vi "test-swerve-drve-odometry-02.vi"() -> (3 "Test Passed":bool)   [LabVIEW 2019]
uses:
  <vilib>/Rock Robotics/WPI/ThirdParty/JAS_Junk/TrajLib/TypeDef/SWERVE_DRIVE_ODOMETRY.ctl
  <vilib>/Rock Robotics/WPI/ThirdParty/JAS_Junk/TrajLib/TypeDef/POSE2D.ctl
  <vilib>/Rock Robotics/WPI/ThirdParty/JAS_Junk/TrajLib/TypeDef/TRANSLATION2D.ctl
  <vilib>/Rock Robotics/WPI/ThirdParty/JAS_Junk/TrajLib/TypeDef/ROTATION2D.ctl
  <vilib>/Rock Robotics/WPI/ThirdParty/JAS_Junk/TrajLib/TypeDef/SWERVE_DRIVE_MODULE_POSITION.ctl
  <vilib>/Rock Robotics/WPI/ThirdParty/JAS_Junk/TrajLib/TypeDef/SWERVE_DRIVE_KINEMATICS.ctl
  <vilib>/Analysis/Matrix/Datatypes/RealMatrix.ctl
  <vilib>/Rock Robotics/WPI/ThirdParty/JAS_Junk/TrajLib/TypeDef/SWERVE_DRIVE_MODULE_STATE.ctl
  <vilib>/Rock Robotics/WPI/ThirdParty/JAS_Junk/TrajLib/Conv_Deg_Radians.vi
  <vilib>/Rock Robotics/WPI/ThirdParty/JAS_Junk/TrajLib/Rotation2d_CreateAngle.vi
  <vilib>/Rock Robotics/WPI/ThirdParty/JAS_Junk/TrajLib/Trajectory_Library.lvlib
  <vilib>/Analysis/Matrix/NI_Matrix.lvlib
panel:
  out "SWERVE_DRIVE_KINEMATICS":T1 {"SavedModuleStates"."Angle"."SIN" format="%13.4f"; "SavedModuleStates"."Angle"."COS" format="%13.4f"; "SavedModuleStates"."Angle"."VALUE" format="%13.4f"; "PrevCoR"."Y" format="%14.3f"; "PrevCoR"."X" format="%14.3f"; "Modules"."Y" format="%14.3f"; "Modules"."X" format="%14.3f"}
  out "Odom 1":T6={"POSE"={"TRANSLATION"={"X"=0.0, "Y"=0.0}, "ROTATION"={"VALUE"=0.0, "COS"=1.0, "SIN"=0.0}}, "GyroOffset"={"VALUE"=0.0, "COS"=1.0, "SIN"=0.0}, "PreviousAngle"={"VALUE"=0.0, "COS"=1.0, "SIN"=0.0}, "PrevModulePositions"=[], "NumModules"=0} {"PrevModulePositions"."Angle"."SIN" format="%13.4f"; "PrevModulePositions"."Angle"."COS" format="%13.4f"; "PrevModulePositions"."Angle"."VALUE" format="%13.4f"; "PreviousAngle"."SIN" format="%13.4f"; "PreviousAngle"."COS" format="%13.4f"; "PreviousAngle"."VALUE" format="%13.4f"; "GyroOffset"."SIN" format="%13.4f"; "GyroOffset"."COS" format="%13.4f"; "GyroOffset"."VALUE" format="%13.4f"; "POSE"."ROTATION"."SIN" format="%13.4f"; "POSE"."ROTATION"."COS" format="%13.4f"; "POSE"."ROTATION"."VALUE" format="%13.4f"; "POSE"."TRANSLATION"."Y" format="%14.3f"; "POSE"."TRANSLATION"."X" format="%14.3f"}
  out "Odom 0":T6={"POSE"={"TRANSLATION"={"X"=0.0, "Y"=0.0}, "ROTATION"={"VALUE"=0.0, "COS"=1.0, "SIN"=0.0}}, "GyroOffset"={"VALUE"=0.0, "COS"=1.0, "SIN"=0.0}, "PreviousAngle"={"VALUE"=0.0, "COS"=1.0, "SIN"=0.0}, "PrevModulePositions"=[], "NumModules"=0} {"PrevModulePositions"."Angle"."SIN" format="%13.4f"; "PrevModulePositions"."Angle"."COS" format="%13.4f"; "PrevModulePositions"."Angle"."VALUE" format="%13.4f"; "PreviousAngle"."SIN" format="%13.4f"; "PreviousAngle"."COS" format="%13.4f"; "PreviousAngle"."VALUE" format="%13.4f"; "GyroOffset"."SIN" format="%13.4f"; "GyroOffset"."COS" format="%13.4f"; "GyroOffset"."VALUE" format="%13.4f"; "POSE"."ROTATION"."SIN" format="%13.4f"; "POSE"."ROTATION"."COS" format="%13.4f"; "POSE"."ROTATION"."VALUE" format="%13.4f"; "POSE"."TRANSLATION"."Y" format="%14.3f"; "POSE"."TRANSLATION"."X" format="%14.3f"}
  out "robot POSE 0":T7={"TRANSLATION"={"X"=0.0, "Y"=0.0}, "ROTATION"={"VALUE"=0.0, "COS"=1.0, "SIN"=0.0}} {"ROTATION"."SIN" format="%13.4f"; "ROTATION"."COS" format="%13.4f"; "ROTATION"."VALUE" format="%13.4f"; "TRANSLATION"."Y" format="%14.3f"; "TRANSLATION"."X" format="%14.3f"}
  out "robot POSE 1":T7={"TRANSLATION"={"X"=0.0, "Y"=0.0}, "ROTATION"={"VALUE"=0.0, "COS"=1.0, "SIN"=0.0}} {"ROTATION"."SIN" format="%13.4f"; "ROTATION"."COS" format="%13.4f"; "ROTATION"."VALUE" format="%13.4f"; "TRANSLATION"."Y" format="%14.3f"; "TRANSLATION"."X" format="%14.3f"}
  out "robot POSE 2":T7={"TRANSLATION"={"X"=0.0, "Y"=0.0}, "ROTATION"={"VALUE"=0.0, "COS"=1.0, "SIN"=0.0}} {"ROTATION"."SIN" format="%13.4f"; "ROTATION"."COS" format="%13.4f"; "ROTATION"."VALUE" format="%13.4f"; "TRANSLATION"."Y" format="%14.3f"; "TRANSLATION"."X" format="%14.3f"}
  out "Odom 2":T6={"POSE"={"TRANSLATION"={"X"=0.0, "Y"=0.0}, "ROTATION"={"VALUE"=0.0, "COS"=1.0, "SIN"=0.0}}, "GyroOffset"={"VALUE"=0.0, "COS"=1.0, "SIN"=0.0}, "PreviousAngle"={"VALUE"=0.0, "COS"=1.0, "SIN"=0.0}, "PrevModulePositions"=[], "NumModules"=0} {"PrevModulePositions"."Angle"."SIN" format="%13.4f"; "PrevModulePositions"."Angle"."COS" format="%13.4f"; "PrevModulePositions"."Angle"."VALUE" format="%13.4f"; "PreviousAngle"."SIN" format="%13.4f"; "PreviousAngle"."COS" format="%13.4f"; "PreviousAngle"."VALUE" format="%13.4f"; "GyroOffset"."SIN" format="%13.4f"; "GyroOffset"."COS" format="%13.4f"; "GyroOffset"."VALUE" format="%13.4f"; "POSE"."ROTATION"."SIN" format="%13.4f"; "POSE"."ROTATION"."COS" format="%13.4f"; "POSE"."ROTATION"."VALUE" format="%13.4f"; "POSE"."TRANSLATION"."Y" format="%14.3f"; "POSE"."TRANSLATION"."X" format="%14.3f"}
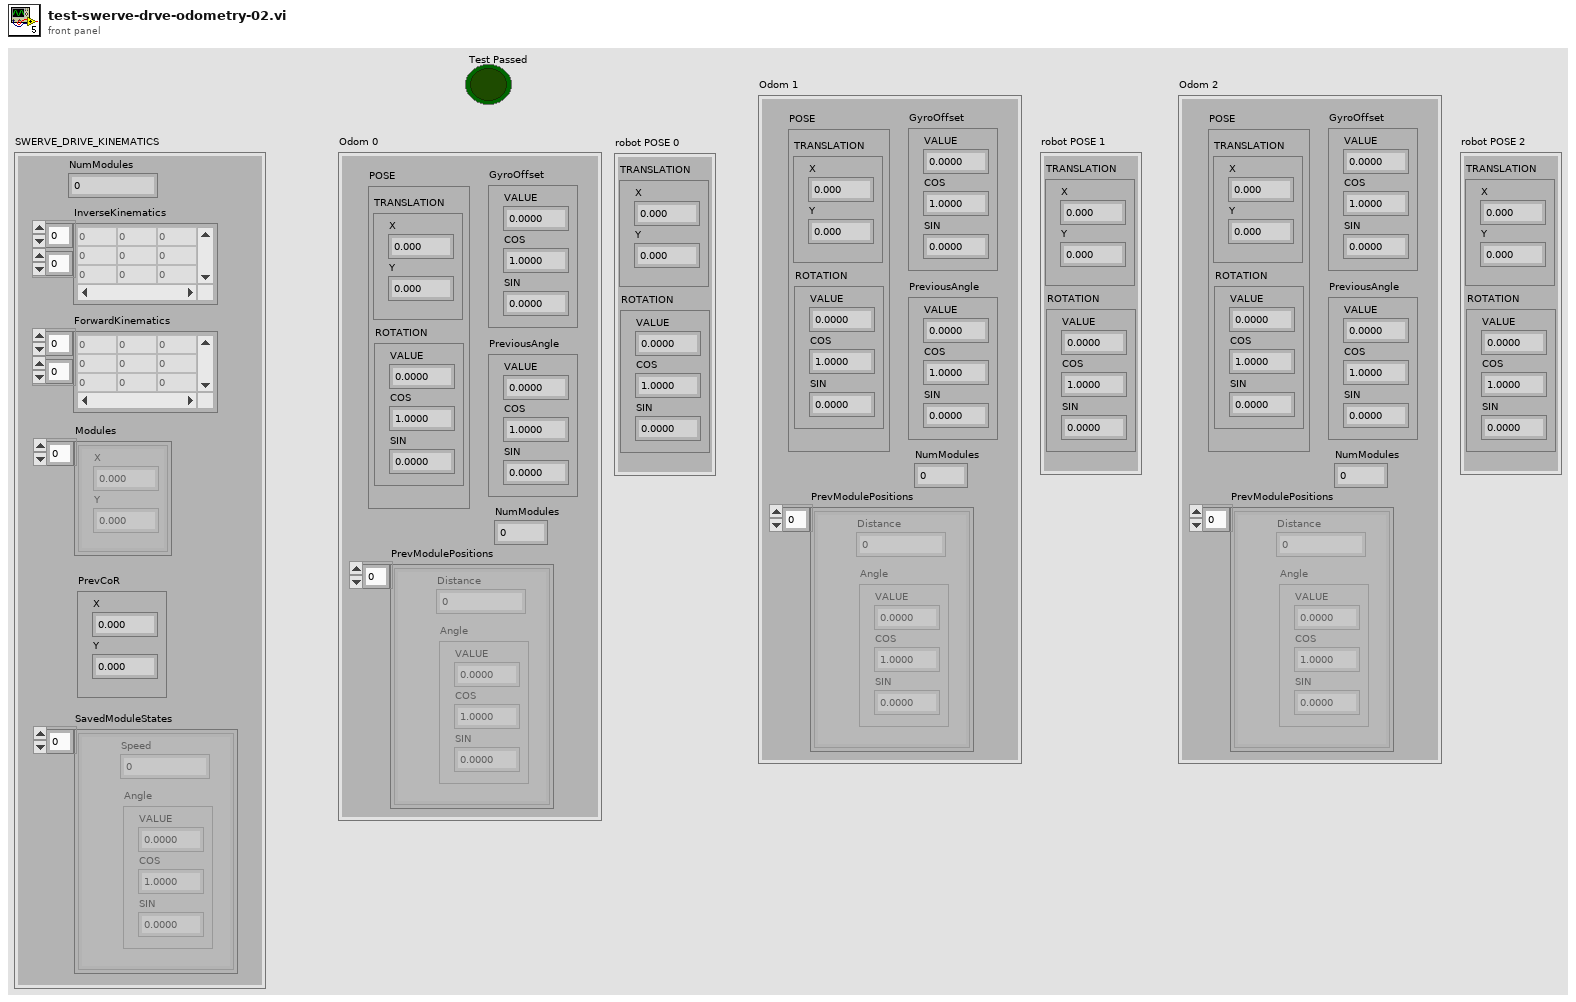
[diagram p1: front panel]
types:
  T1 = typedef "Trajectory_Library.lvlib/SWERVE_DRIVE_KINEMATICS.ctl" = cluster{"NumModules":i32, "InverseKinematics":T2, "ForwardKinematics":T2, "Modules":T3[], "PrevCoR":T3, "SavedModuleStates":T4[]}
  T2 = typedef "NI_Matrix.lvlib/RealMatrix.ctl" = dbl[][]
  T3 = typedef "Trajectory_Library.lvlib/TRANSLATION2D.ctl" = cluster{"X":dbl, "Y":dbl}
  T4 = typedef "Trajectory_Library.lvlib/SWERVE_DRIVE_MODULE_STATE.ctl" = cluster{"Speed":dbl, "Angle":T5}
  T5 = typedef "Trajectory_Library.lvlib/ROTATION2D.ctl" = cluster{"VALUE":dbl, "COS":dbl, "SIN":dbl}
  T6 = typedef "Trajectory_Library.lvlib/SWERVE_DRIVE_ODOMETRY.ctl" = cluster{"POSE":T7, "GyroOffset":T5, "PreviousAngle":T5, "PrevModulePositions":T8[], "NumModules":i32}
  T7 = typedef "Trajectory_Library.lvlib/POSE2D.ctl" = cluster{"TRANSLATION":T3, "ROTATION":T5}
  T8 = typedef "Trajectory_Library.lvlib/SWERVE_DRIVE_MODULE_POSITION.ctl" = cluster{"Distance":dbl, "Angle":T5}
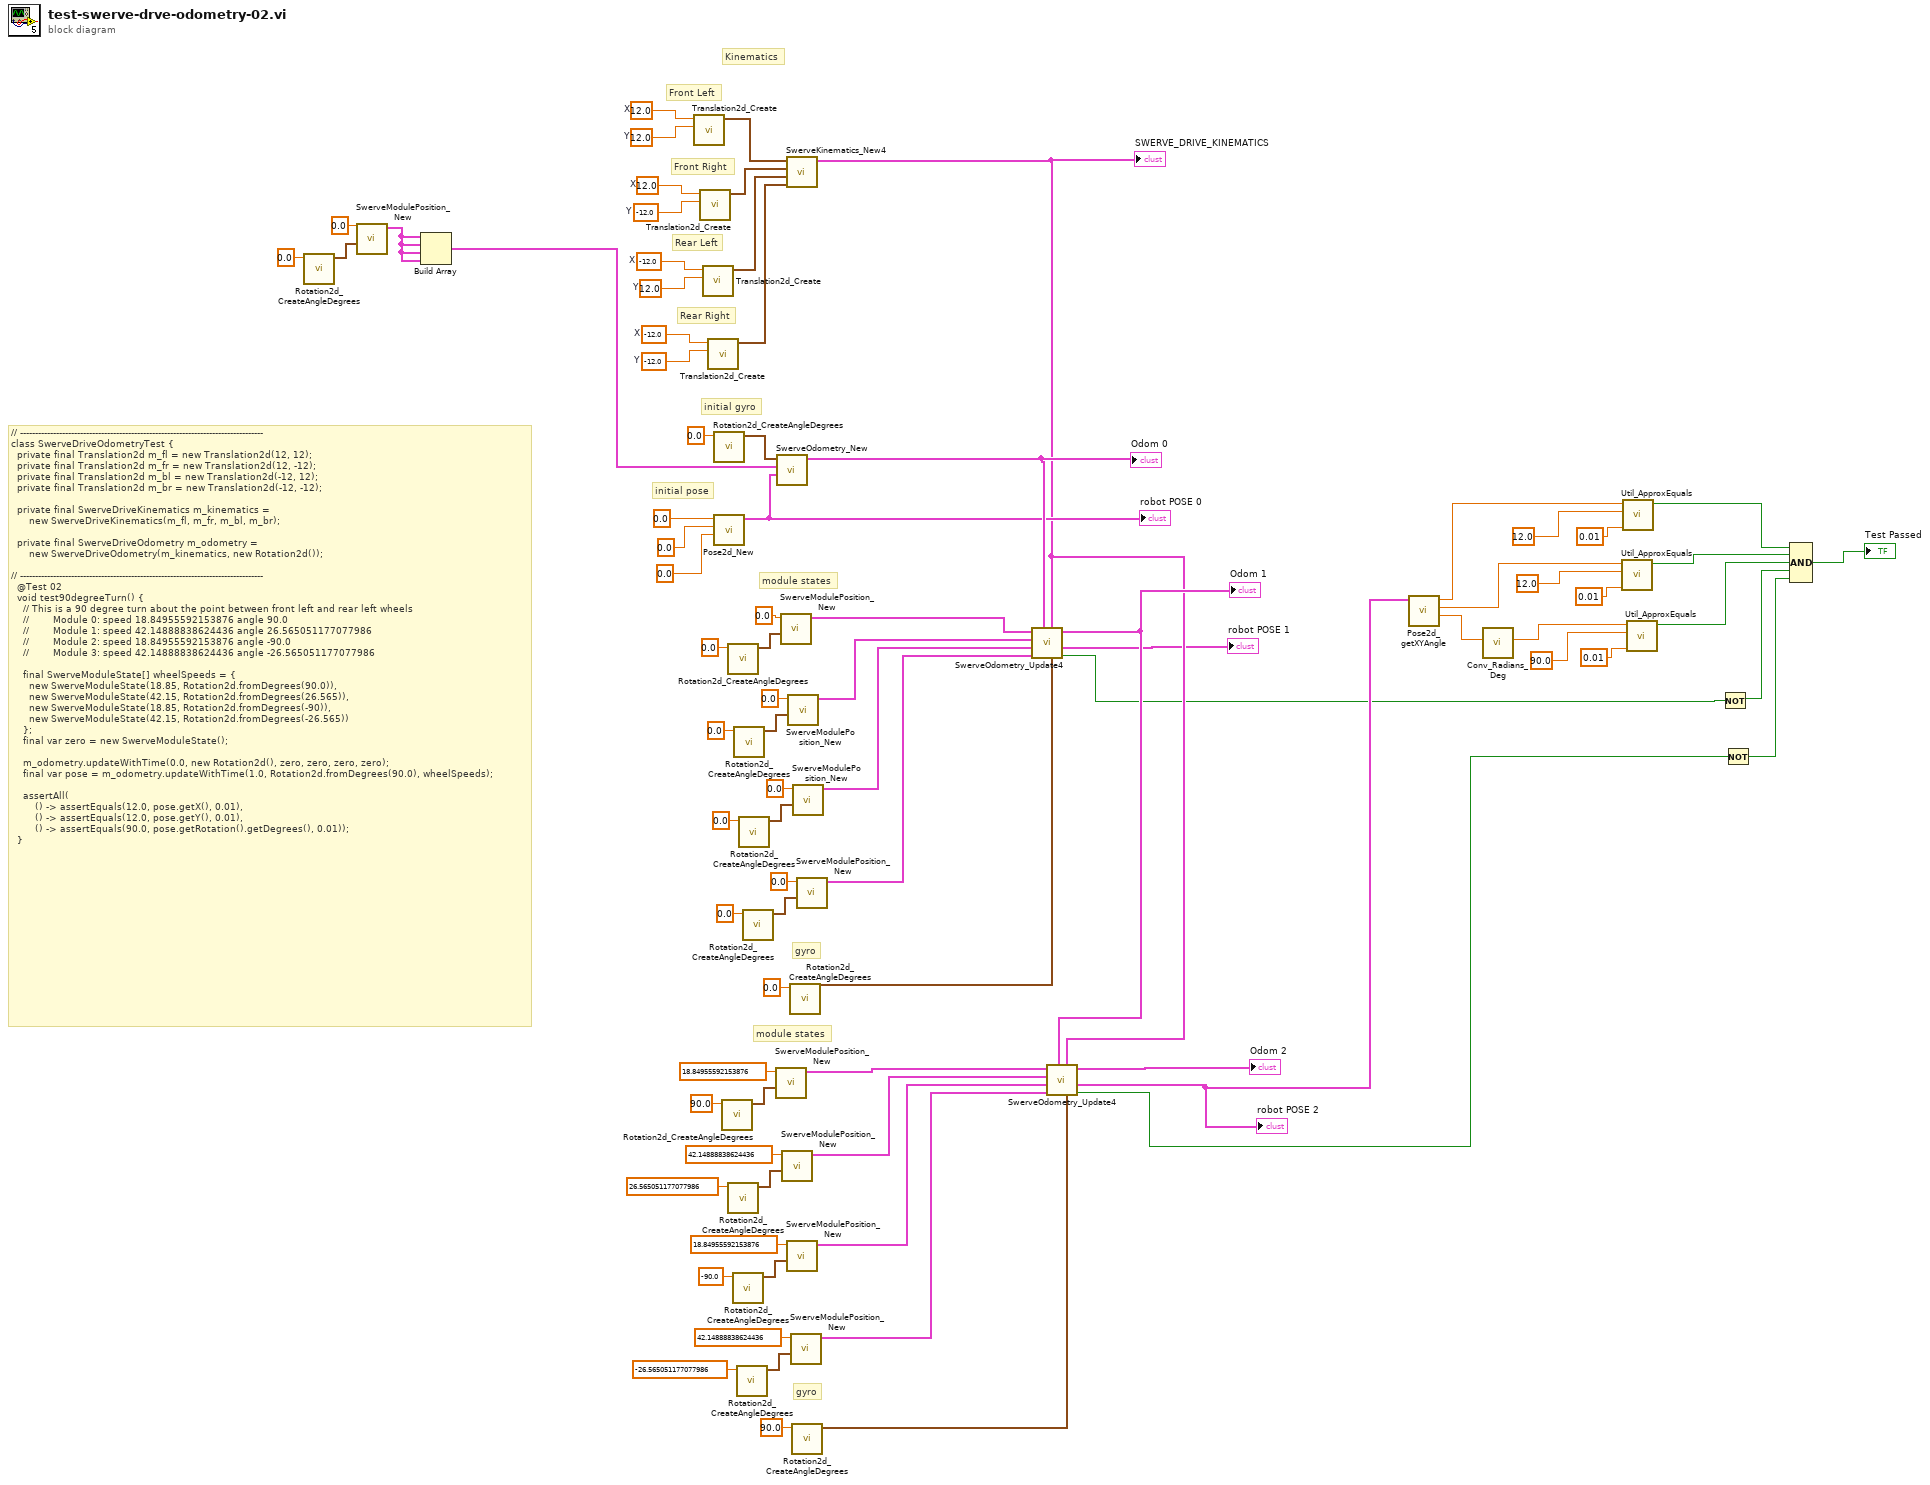
[diagram p0: block diagram]
diagram:
  w79 = -12.0  # X
  w78 = -12.0  # Y
  w77 = -12.0  # X
  w76 = 12.0  # Y
  w75 = 12.0  # X
  w74 = -12.0  # Y
  w73 = 12.0  # X
  w72 = 12.0  # Y
  # "initial pose"
  # "gyro"
  # "module states"
  # "gyro"
  # "module states"
  # "Kinematics"
  # "initial gyro"
  # "Rear Right"
  # "Rear Left"
  # "Front Right"
  # "Front Left"
  # "// ---------------------------------------------------------------------------------\nclass SwerveDriveOdometryTest {\n  private final Translation2d m_fl = new Translation2d(12, 12);\n  private final Translation2d m_fr = new Translation2d(12, -12);\n  private final Translation2d m_bl = new Translation2d(-12, 12);\n  private final Translation2d m_br = new Translation2d(-12, -12);\n\n  private final SwerveDriveKinematics m_kinematics =\n      new SwerveDriveKinematics(m_fl, m_fr, m_bl, m_br);\n\n  private final SwerveDriveOdometry m_odometry =\n      new SwerveDriveOdometry(m_kinematics, new Rotation2d());\n\n// ---------------------------------------------------------------------------------\n  @Test 02\n  void test90degreeTurn() {\n    // This is a 90 degree turn about the point between front left and rear left wheels\n    //        Module 0: speed 18.84955592153876 angle 90.0\n    //        Module 1: speed 42.14888838624436 angle 26.565051177077986\n    //        Module 2: speed 18.84955592153876 angle -90.0\n    //        Module 3: speed 42.14888838624436 angle -26.565051177077986\n\n    final SwerveModuleState[] wheelSpeeds = {\n      new SwerveModuleState(18.85, Rotation2d.fromDegrees(90.0)),\n      new SwerveModuleState(42.15, Rotation2d.fromDegrees(26.565)),\n      new SwerveModuleState(18.85, Rotation2d.fromDegrees(-90)),\n      new SwerveModuleState(42.15, Rotation2d.fromDegrees(-26.565))\n    };\n    final var zero = new SwerveModuleState();\n\n    m_odometry.updateWithTime(0.0, new Rotation2d(), zero, zero, zero, zero);\n    final var pose = m_odometry.updateWithTime(1.0, Rotation2d.fromDegrees(90.0), wheelSpeeds);\n\n    assertAll(\n        () -> assertEquals(12.0, pose.getX(), 0.01),\n        () -> assertEquals(12.0, pose.getY(), 0.01),\n        () -> assertEquals(90.0, pose.getRotation().getDegrees(), 0.01));\n  }"
  n1 = call <vilib>:"Rotation2d_CreateAngleDegrees.vi"("Angle_Degrees"=0.0) -> ("ROTATION"=w8:T5)  [unwired: 10 in]
  n2 = call <vilib>:"SwerveModulePosition_New.vi"("ROTATION"=w8, "Distance"=0.0 ("Speed")) -> ("SWERVE_DRIVE_MODULE_POSITION"=w6:T8)  [unwired: 9 in]
  n3 = Build Array(w6, w6, w6, w6) -> (w5:T8[])
  n4 = call <vilib>:"Translation2d_Create.vi"("Y"=w72, "X"=w73) -> ("TRANSLATION"=w80:T3)  [unwired: 9 in]
  n5 = call <vilib>:"Translation2d_Create.vi"("Y"=w74, "X"=w75) -> ("TRANSLATION"=w81:T3)  [unwired: 9 in]
  n6 = call <vilib>:"Translation2d_Create.vi"("Y"=w76, "X"=w77) -> ("TRANSLATION"=w82:T3)  [unwired: 9 in]
  n7 = call <vilib>:"Translation2d_Create.vi"("Y"=w78, "X"=w79) -> ("TRANSLATION"=w83:T3)  [unwired: 9 in]
  n8 = call <vilib>:"Rotation2d_CreateAngleDegrees.vi"("Angle_Degrees"=0.0) -> ("ROTATION"=w68:T5)  [unwired: 10 in]
  n9 = call <vilib>:"Pose2d_New.vi"("Heading"=0.0, "Y"=0.0, "X"=0.0) -> ("out POSe"=w37:T7)  [unwired: 8 in]
  "robot POSE 0" <- w37
  n10 = call <vilib>:"Rotation2d_CreateAngleDegrees.vi"("Angle_Degrees"=90.0) -> ("ROTATION"=w65:T5)  [unwired: 10 in]
  n11 = call <vilib>:"Rotation2d_CreateAngleDegrees.vi"("Angle_Degrees"=0.0) -> ("ROTATION"=w53:T5)  [unwired: 10 in]
  n12 = call <vilib>:"Rotation2d_CreateAngleDegrees.vi"("Angle_Degrees"=26.565051177077986) -> ("ROTATION"=w62:T5)  [unwired: 10 in]
  n13 = call <vilib>:"Rotation2d_CreateAngleDegrees.vi"("Angle_Degrees"=-90.0) -> ("ROTATION"=w59:T5)  [unwired: 10 in]
  n14 = call <vilib>:"Rotation2d_CreateAngleDegrees.vi"("Angle_Degrees"=0.0) -> ("ROTATION"=w50:T5)  [unwired: 10 in]
  n15 = call <vilib>:"Rotation2d_CreateAngleDegrees.vi"("Angle_Degrees"=-26.565051177077986) -> ("ROTATION"=w56:T5)  [unwired: 10 in]
  n16 = call <vilib>:"Rotation2d_CreateAngleDegrees.vi"("Angle_Degrees"=0.0) -> ("ROTATION"=w47:T5)  [unwired: 10 in]
  n17 = call <vilib>:"Rotation2d_CreateAngleDegrees.vi"("Angle_Degrees"=0.0) -> ("ROTATION"=w44:T5)  [unwired: 10 in]
  n18 = call <vilib>:"SwerveModulePosition_New.vi"("ROTATION"=w65, "Distance"=18.84955592153876 ("Speed")) -> ("SWERVE_DRIVE_MODULE_POSITION"=w13:T8)  [unwired: 9 in]
  n19 = call <vilib>:"SwerveOdometry_New.vi"("InitialPose"=w37, "Module Positions"=w5, "gyroAngle"=w68) -> ("SWERVE_DRIVE_ODOMETRY"=w38:T6)  [unwired: 8 in]
  "Odom 0" <- w38
  n20 = call <vilib>:"SwerveModulePosition_New.vi"("ROTATION"=w53, "Distance"=0.0 ("Speed")) -> ("SWERVE_DRIVE_MODULE_POSITION"=w17:T8)  [unwired: 9 in]
  n21 = call <vilib>:"SwerveModulePosition_New.vi"("ROTATION"=w62, "Distance"=42.14888838624436 ("Speed")) -> ("SWERVE_DRIVE_MODULE_POSITION"=w12:T8)  [unwired: 9 in]
  n22 = call <vilib>:"SwerveKinematics_New4.vi"("wheel 3"=w83, "wheel 2"=w82, "wheel 1"=w81, "wheel 0"=w80) -> ("SWERVE_DRIVE_KINEMATICS"=w34:T1)  [unwired: 7 in]
  "SWERVE_DRIVE_KINEMATICS" <- w34
  n23 = call <vilib>:"SwerveModulePosition_New.vi"("ROTATION"=w59, "Distance"=18.84955592153876 ("Speed")) -> ("SWERVE_DRIVE_MODULE_POSITION"=w11:T8)  [unwired: 9 in]
  n24 = call <vilib>:"SwerveModulePosition_New.vi"("ROTATION"=w50, "Distance"=0.0 ("Speed")) -> ("SWERVE_DRIVE_MODULE_POSITION"=w16:T8)  [unwired: 9 in]
  n25 = call <vilib>:"Rotation2d_CreateAngleDegrees.vi"("Angle_Degrees"=0.0) -> ("ROTATION"=w41:T5)  [unwired: 10 in]
  n26 = call <vilib>:"SwerveModulePosition_New.vi"("ROTATION"=w56, "Distance"=42.14888838624436 ("Speed")) -> ("SWERVE_DRIVE_MODULE_POSITION"=w10:T8)  [unwired: 9 in]
  n27 = call <vilib>:"Rotation2d_CreateAngleDegrees.vi"("Angle_Degrees"=90.0) -> ("ROTATION"=w39:T5)  [unwired: 10 in]
  n28 = call <vilib>:"SwerveModulePosition_New.vi"("ROTATION"=w47, "Distance"=0.0 ("Speed")) -> ("SWERVE_DRIVE_MODULE_POSITION"=w15:T8)  [unwired: 9 in]
  n29 = call <vilib>:"SwerveModulePosition_New.vi"("ROTATION"=w44, "Distance"=0.0 ("Speed")) -> ("SWERVE_DRIVE_MODULE_POSITION"=w14:T8)  [unwired: 9 in]
  n30 = call <vilib>:"SwerveOdometry_Update4.vi"("gyroAngle"=w41, "SWERVE_DRIVE_KINEMATICS"=w34, "in SWERVE_DRIVE_ODOMETRY"=w38, "Wheel Position 3"=w14, "Wheel Position 2"=w15, "Wheel Position 1"=w16, "Wheel Position 0"=w17) -> ("Error"=w4:bool, "robot POSE"=→"robot POSE 1":T7, "out SWERVE_DRIVE_ODOMETRY"=w36:T6)  [unwired: 2 in]
  "Odom 1" <- w36
  n31 = call <vilib>:"SwerveOdometry_Update4.vi"("gyroAngle"=w39, "SWERVE_DRIVE_KINEMATICS"=w34, "in SWERVE_DRIVE_ODOMETRY"=w36, "Wheel Position 3"=w10, "Wheel Position 2"=w11, "Wheel Position 1"=w12, "Wheel Position 0"=w13) -> ("Error"=w3:bool, "robot POSE"=w18:T7, "out SWERVE_DRIVE_ODOMETRY"=→"Odom 2":T6)  [unwired: 2 in]
  "robot POSE 2" <- w18
  n32 = call <vilib>:"Pose2d_getXYAngle.vi"("in POSE"=w18) -> ("Angle"=w30:dbl, "Y"=w27:dbl, "X"=w28:dbl)  [unwired: 8 in]
  n33 = call <vilib>:"Conv_Radians_Deg.vi"("Radians"=w30) -> ("Degrees"=w26:dbl)  [unwired: 10 in]
  n34 = call <vilib>:"Util_ApproxEquals.vi"("Tolerance"=0.01, "Value 2"=12.0, "Value 1"=w27) -> ("ApproxEquals"=w21:bool)  [unwired: 8 in]
  n35 = call <vilib>:"Util_ApproxEquals.vi"("Tolerance"=0.01, "Value 2"=12.0, "Value 1"=w28) -> ("ApproxEquals"=w22:bool)  [unwired: 8 in]
  n36 = call <vilib>:"Util_ApproxEquals.vi"("Tolerance"=0.01, "Value 2"=90.0, "Value 1"=w26) -> ("ApproxEquals"=w20:bool)  [unwired: 8 in]
  n37 = Not(x=w4) -> (.not. x?=w2:bool)
  n38 = Not(x=w3) -> (.not. x?=w1:bool)
  n39 = Compound Arithmetic op=AND(w22, w21, w20, w2, w1) -> (→"Test Passed":bool)
